vi "WrongDateFormatCorrect.vi"(10 "String":string) -> (2 "concatenated string":string)   [LabVIEW 2012]
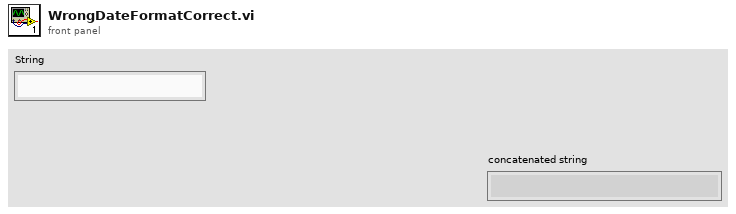
[diagram p1: front panel]
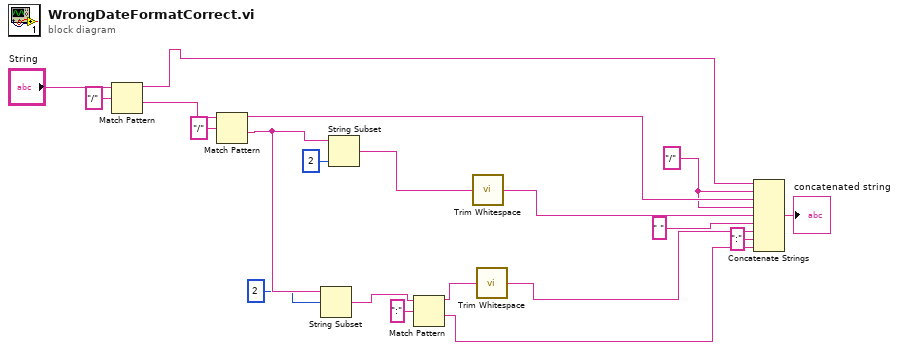
[diagram p0: block diagram]
diagram:
  w9 = "/" ("string")
  n1 = Match Pattern(string="String", regular expression="/") -> (before substring=w11:string, after substring=w17:string)  [unwired: 1 in, 2 out]
  n2 = Match Pattern(string=w17, regular expression="/") -> (before substring=w10:string, after substring=w15:string)  [unwired: 1 in, 2 out]
  n3 = String Subset(string=w15, offset (0)=2) -> (substring=w12:string)  [unwired: 1 in]
  n4 = String Subset(string=w15, length (rest)=2 ("length (rest)")) -> (substring=w1:string)  [unwired: 1 in]
  n5 = Match Pattern(string=w12, regular expression=":") -> (before substring=w3:string, after substring=w6:string)  [unwired: 1 in, 2 out]
  n6 = call <vilib>:"Trim Whitespace.vi"("string"=w1) -> ("trimmed string"=w2:string)  [unwired: 1 in]
  n7 = call <vilib>:"Trim Whitespace.vi"("string"=w3) -> ("trimmed string"=w4:string)  [unwired: 1 in]
  n8 = Concatenate Strings(w11, w9, w10, w9, w2, " " ("string"), w4, ":" ("string"), w6) -> (→"concatenated string":string)
